vi "Host_ShVariables.vi"() -> ()   [LabVIEW 2019]
panel:
  in  "stop":bool
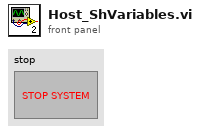
[diagram p1: front panel]
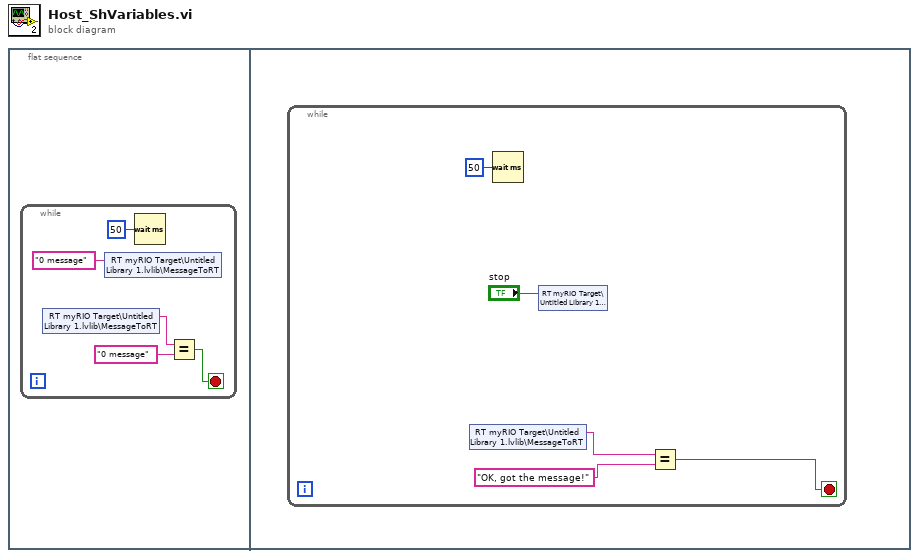
[diagram p0: block diagram]
diagram:
  n1 = flat-sequence {
    frame #0 {
      n2 = while {
        stop <- w2 stop-if-true
        n3 = shared-variable "RT myRIO Target\\Untitled Library 1.lvlib\\MessageToRT"() -> (w4:string)  [unwired: 1 in, 1 out]
        n4 = shared-variable "RT myRIO Target\\Untitled Library 1.lvlib\\MessageToRT"("0 message" ("MessageToRT")) -> ()  [unwired: 1 in, 1 out]
        n5 = Wait (ms)(milliseconds to wait=u32 50) -> ()  [unwired: 1 out]
        n6 = Equal?(x=w4, y="0 message") -> (x = y?=w2:bool)
      }
    }
    frame #1 {
      n7 = while {
        stop <- w7 stop-if-true
        n8 = shared-variable "RT myRIO Target\\Untitled Library 1.lvlib\\MessageToRT"() -> (w9:string)  [unwired: 1 in, 1 out]
        n9 = Wait (ms)(milliseconds to wait=u32 50) -> ()  [unwired: 1 out]
        n10 = shared-variable "RT myRIO Target\\Untitled Library 1.lvlib\\Stop"("stop") -> ()  [unwired: 1 in, 1 out]
        n11 = Equal?(x=w9, y="OK, got the message!") -> (x = y?=w7:bool)
      }
    }
  }
